vi "PIV_Cell_Selector.vi"(11 "CHC":dbl[][](array[numeric])) -> (1 "Y Index":i32, 2 "X Index":i32)   [LabVIEW 2011]
panel:
  out "CHC":dbl[][](graph)
  in  "OK Button":bool
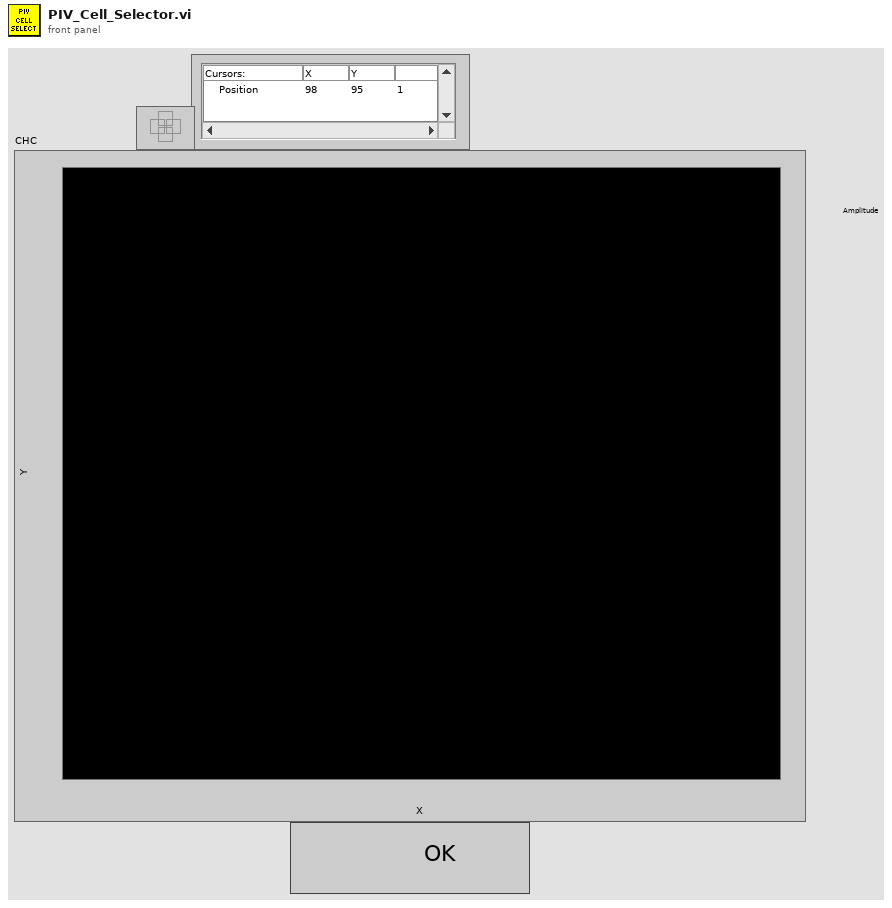
[diagram p1: front panel]
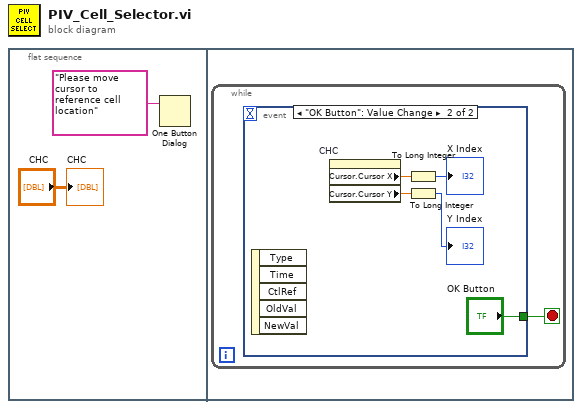
[diagram p0: block diagram]
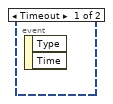
[diagram p2: hidden frame]
diagram:
  n1 = flat-sequence {
    frame #0 {
      n2 = One Button Dialog(message="Please move cursor to reference cell location") -> ()  [unwired: 1 in, 1 out]
      "CHC" <- "CHC"
    }
    frame #1 {
      n3 = while {
        stop <- w3 stop-if-true
        n4 = event shown="[1] \"OK Button\": Value Change" {
          selector: _ -> [_ _]
          dyn-events: _ -> [_ _]
          timeout: _ -> [_ _]
          tunnel: [_ "OK Button"] -> w3
          event Timeout {
            n5 = event-data() -> ()  [unwired: 1 in, 2 out]
          }
          event "OK Button": Value Change {
            n6 = event-data() -> ()  [unwired: 1 in, 5 out]
            n7 = property on="CHC" class="IntGraph (strict)"() -> ("Cursor.Cursor X"=w7:dbl, "Cursor.Cursor Y"=w5:dbl)  [unwired: 2 in, 2 out]
            n8 = To Long Integer(number=w7) -> (32bit integer=→"X Index":i32)
            n9 = To Long Integer(number=w5) -> (32bit integer=→"Y Index":i32)
          }
        }
      }
    }
  }
